vi "test-ElevatorSim-stability.vi"() -> (3 "Test Passed":bool)   [LabVIEW 2019]
uses:
  <vilib>/Rock Robotics/WPI/ThirdParty/JAS_Junk/TrajLib/TypeDef/DCMOTOR.CTL
  <vilib>/Rock Robotics/WPI/ThirdParty/JAS_Junk/TrajLib/TypeDef/ELEVATOR_SIM.ctl
  <vilib>/Rock Robotics/WPI/ThirdParty/JAS_Junk/TrajLib/TypeDef/LINEAR_SYSTEM_SIM.ctl
  <vilib>/Rock Robotics/WPI/ThirdParty/JAS_Junk/TrajLib/TypeDef/LINEAR_SYSTEM.ctl
  <vilib>/Analysis/Matrix/Datatypes/RealMatrix.ctl
  <vilib>/Rock Robotics/WPI/ThirdParty/JAS_Junk/TrajLib/MatBuilder_Create.vi
  <vilib>/Rock Robotics/WPI/ThirdParty/JAS_Junk/TrajLib/DCMotor_New.vi
  <vilib>/Rock Robotics/WPI/ThirdParty/JAS_Junk/TrajLib/VI/Units_RotationsPerMinuteToRadiansPerSecond.vi
  <vilib>/Rock Robotics/WPI/ThirdParty/JAS_Junk/TrajLib/Discretization_DiscretizeAB.vi
  <vilib>/Analysis/baseanly.llb/A x B.vi
  <vilib>/Analysis/baseanly.llb/Real A x B.vi
  <vilib>/Rock Robotics/WPI/ThirdParty/JAS_Junk/TrajLib/MatrixHelper_CoerceSize.vi
  <vilib>/Rock Robotics/WPI/ThirdParty/JAS_Junk/TrajLib/Matrix_Exp.vi
  <vilib>/Rock Robotics/WPI/ThirdParty/JAS_Junk/TrajLib/Matrix_AssignBlock.vi
  <vilib>/Rock Robotics/WPI/ThirdParty/JAS_Junk/TrajLib/Matrix_ExtractFrom.vi
  <vilib>/Analysis/7linalg.llb/Matrix Exp.vi
  <vilib>/Analysis/7linalg.llb/Real Matrix Exp.vi
  <vilib>/Analysis/Matrix/Numeric/Multiply/Multiply.vi
  <vilib>/Analysis/Matrix/Numeric/Multiply/Multiply - RM,R.vi
  <vilib>/Analysis/Matrix/Numeric/Add/Add.vi
  <vilib>/Analysis/Matrix/Numeric/Add/Add - RM,RM.vi
  <vilib>/Rock Robotics/WPI/ThirdParty/JAS_Junk/TrajLib/Trajectory_Library.lvlib
  <vilib>/Analysis/Matrix/NI_Matrix.lvlib
panel:
  in  "Tab Control":enum32{"Page 2", "Page 6", "Page 7"}(tab)
  out "Elevator Motor":T1 {"Jr_KgM2" format="%13.5p"; "L_H" format="%13.5p"; "Kt_NMPerAmp" format="%13.5p"; "KvINV_RadPerSecPerVolt" format="%13.5p"; "R_Ohms" format="%13.5p"; "FreeSpeed_RadPerSec" format="%13.5p"; "FreeCurrent_Amps" format="%13.5p"; "StallCurrent_Amps" format="%13.5p"; "StallTorque_NM" format="%13.5p"; "nominalVoltage_Volts" format="%13.5p"}
  out "Elevator Simulaation":T2={"LinearSystemSim"={"m_Plant"={"m_A"=[], "m_B"=[], "m_C"=[], "m_D"=[], "States"=0, "Inputs"=0, "Outputs"=0}, "m_X"=[], "m_Y"=[], "m_U"=[], "MeasureStdDev"=[]}, "GearBox"={"nominalVoltage_Volts"=0.0, "StallTorque_NM"=0.0, "StallCurrent_Amps"=0.0, "FreeCurrent_Amps"=0.0, "FreeSpeed_RadPerSec"=0.0, "R_Ohms"=0.0, "KvINV_RadPerSecPerVolt"=0.0, "Kt_NMPerAmp"=0.0, "L_H"=0.0, "Jr_KgM2"=0.0}, "Gearing"=0.0, "DrumRadius_M"=0.0, "MinHeight_M"=0.0, "MaxHeight_M"=0.0, "CarriageMass_Kg"=0.0, "SimulateGravity"=TRUE} {"GearBox"."Jr_KgM2" format="%13.5p"; "GearBox"."L_H" format="%13.5p"; "GearBox"."Kt_NMPerAmp" format="%13.5p"; "GearBox"."KvINV_RadPerSecPerVolt" format="%13.5p"; "GearBox"."R_Ohms" format="%13.5p"; "GearBox"."FreeSpeed_RadPerSec" format="%13.5p"; "GearBox"."FreeCurrent_Amps" format="%13.5p"; "GearBox"."StallCurrent_Amps" format="%13.5p"; "GearBox"."StallTorque_NM" format="%13.5p"; "GearBox"."nominalVoltage_Volts" format="%13.5p"}
  out "Velocity":cluster{"Voltage":dbl}(graph)
  out "PV Chart":cluster{dbl}(graph)
  out "At Top":bool
  out "At Bottom":bool
  out "Size Coerced":bool
  out "Alt Position Meters":dbl
  out "Position_Meters":dbl
  out "ApproxEquals":bool
  # "<States, 1>"
  # "<Outputs, 1>"
  # "<Inputs, 1>"
  # "<Outputs, 1>"
  # "<States,States>"
  # "<States,Inputs>"
  # "<Outputs,States>"
  # "<Outputs,Inputs>"
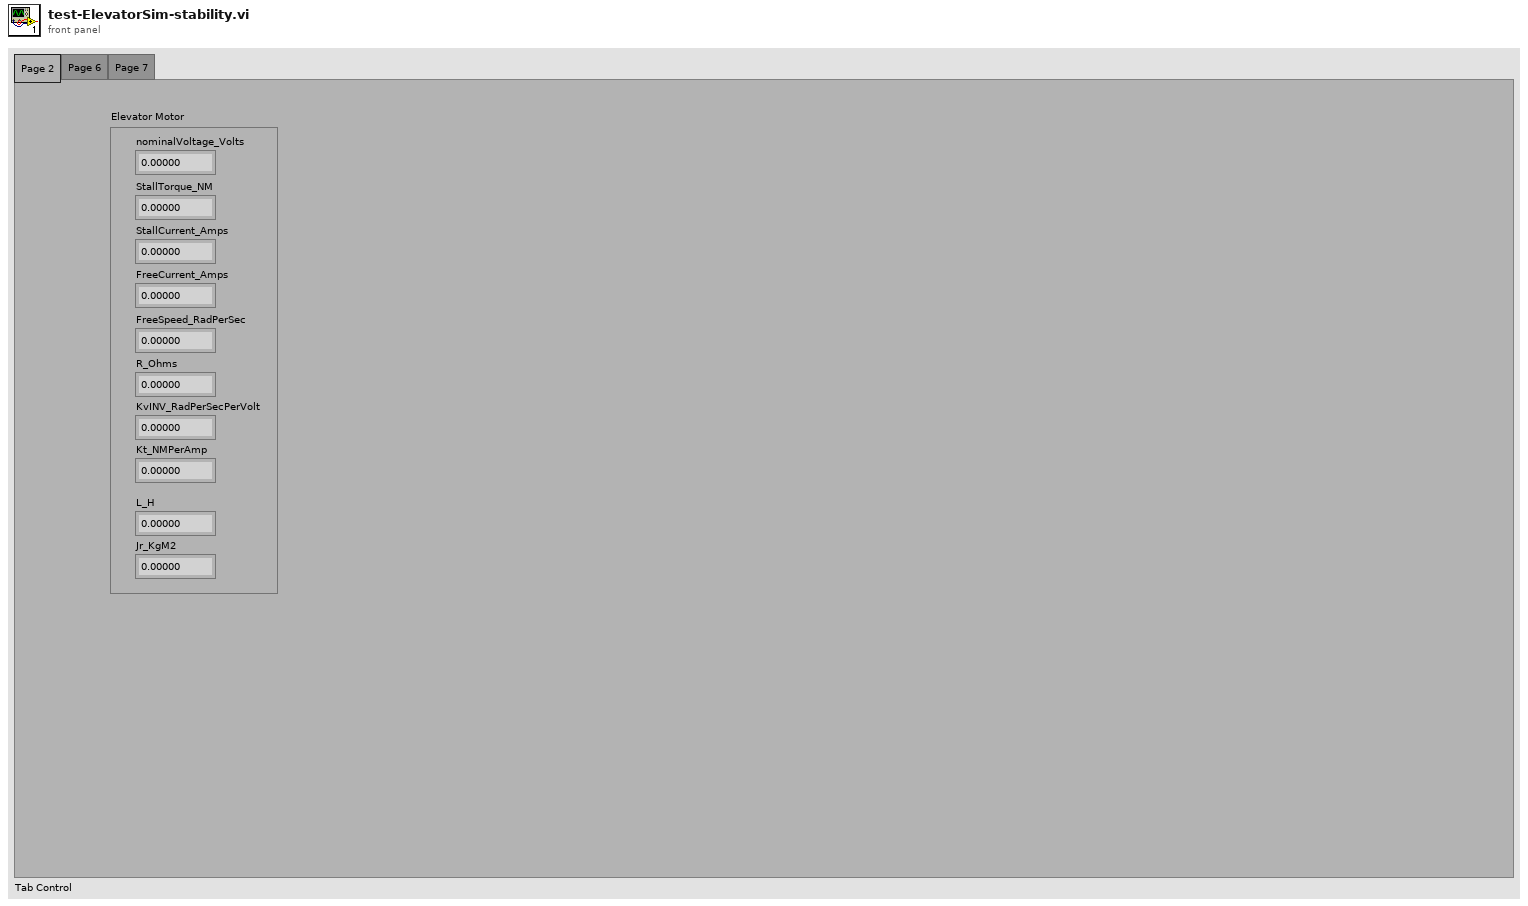
[diagram p1: front panel]
types:
  T1 = typedef "Trajectory_Library.lvlib/DCMOTOR.CTL" = cluster{"nominalVoltage_Volts":dbl, "StallTorque_NM":dbl, "StallCurrent_Amps":dbl, "FreeCurrent_Amps":dbl, "FreeSpeed_RadPerSec":dbl, "R_Ohms":dbl, "KvINV_RadPerSecPerVolt":dbl, "Kt_NMPerAmp":dbl, "L_H":dbl, "Jr_KgM2":dbl}
  T2 = typedef "Trajectory_Library.lvlib/ELEVATOR_SIM.ctl" = cluster{"LinearSystemSim":T3, "GearBox":T1, "Gearing":dbl, "DrumRadius_M":dbl, "MinHeight_M":dbl, "MaxHeight_M":dbl, "CarriageMass_Kg":dbl, "SimulateGravity":bool}
  T3 = typedef "Trajectory_Library.lvlib/LINEAR_SYSTEM_SIM.ctl" = cluster{"m_Plant":T4, "m_X":T5, "m_Y":T5, "m_U":T5, "MeasureStdDev":T5}
  T4 = typedef "Trajectory_Library.lvlib/LINEAR_SYSTEM.ctl" = cluster{"m_A":T5, "m_B":T5, "m_C":T5, "m_D":T5, "States":i32, "Inputs":i32, "Outputs":i32}
  T5 = typedef "NI_Matrix.lvlib/RealMatrix.ctl" = dbl[][]
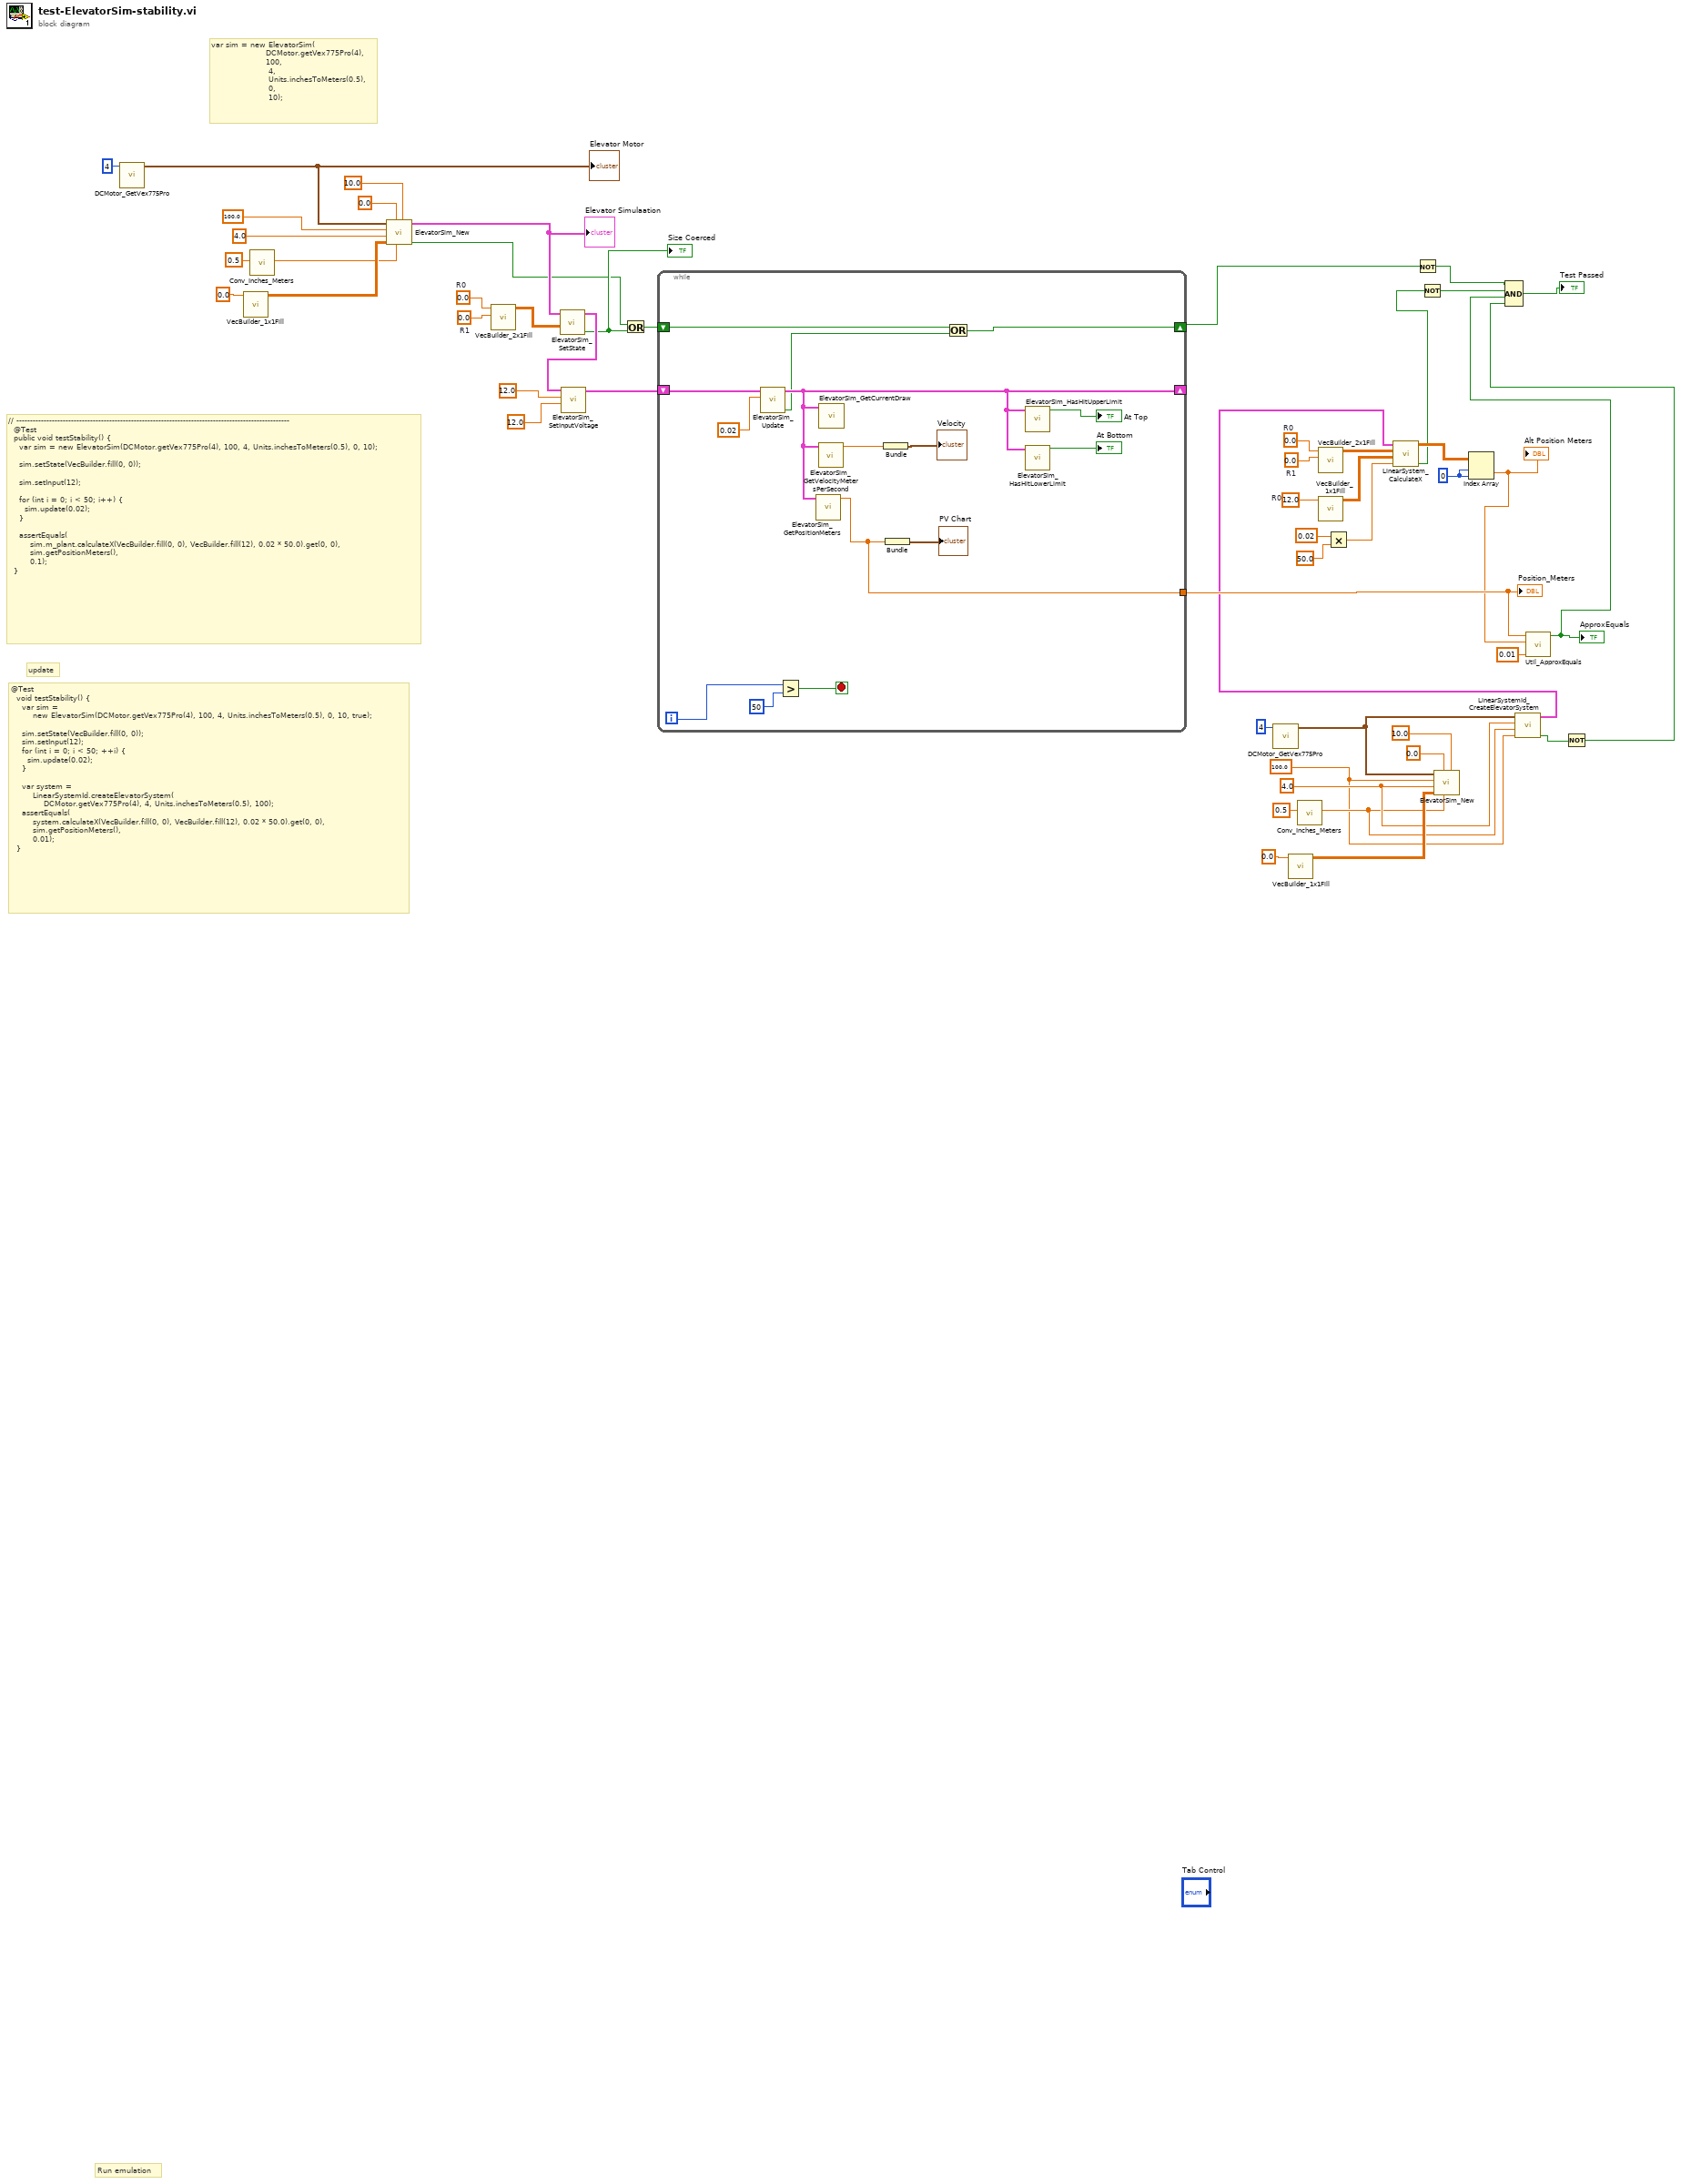
[diagram p0: block diagram]
diagram:
  w4 = 100.0 ("G")
  w6 = 4.0 ("massKg")
  w26 = 0 ("index (row)")
  w33 = 12.0  # R0
  w35 = 0.0  # R1
  w34 = 0.0  # R0
  w38 = 0.0  # R1
  w37 = 0.0  # R0
  # "update"
  # "@Test\n  void testStability() {\n    var sim =\n        new ElevatorSim(DCMotor.getVex775Pro(4), 100, 4, Units.inchesToMeters(0.5), 0, 10, true);\n\n    sim.setState(VecBuilder.fill(0, 0));\n    sim.setInput(12);\n    for (int i = 0; i < 50; ++i) {\n      sim.update(0.02);\n    }\n\n    var system =\n        LinearSystemId.createElevatorSystem(\n            DCMotor.getVex775Pro(4), 4, Units.inchesToMeters(0.5), 100);\n    assertEquals(\n        system.calculateX(VecBuilder.fill(0, 0), VecBuilder.fill(12), 0.02 * 50.0).get(0, 0),\n        sim.getPositionMeters(),\n        0.01);\n  }"
  # "// ----------------------------------------------------------------------------------------------------\n  @Test\n  public void testStability() {\n    var sim = new ElevatorSim(DCMotor.getVex775Pro(4), 100, 4, Units.inchesToMeters(0.5), 0, 10);\n\n    sim.setState(VecBuilder.fill(0, 0));\n\n    sim.setInput(12);\n\n    for (int i = 0; i < 50; i++) {\n      sim.update(0.02);\n    }\n\n    assertEquals(\n        sim.m_plant.calculateX(VecBuilder.fill(0, 0), VecBuilder.fill(12), 0.02 * 50.0).get(0, 0),\n        sim.getPositionMeters(),\n        0.1);\n  }"
  # "var sim = new ElevatorSim(\n                    DCMotor.getVex775Pro(4), \n                    100, \n                     4, \n                     Units.inchesToMeters(0.5), \n                     0, \n                     10);"
  # "Run emulation"
  n1 = call <vilib>:"DCMotor_GetVex775Pro.vi"("Num Motors"=4) -> ("DCMOTOR"=w46:T1)  [unwired: 10 in]
  "Elevator Motor" <- w46
  n2 = call <vilib>:"VecBuilder_1x1Fill.vi"("R0_C0"=0.0) -> ("output matrix"=w50:T5)  [unwired: 10 in]
  n3 = call <vilib>:"Conv_Inches_Meters.vi"("INCH"=0.5) -> ("Meters"=w44:dbl)  [unwired: 10 in]
  n4 = call <vilib>:"ElevatorSim_New.vi"("MaxHeight_Meters"=10.0, "DrumRadius_Meters"=w44, "MinHeight_Meters"=0.0, "MeasurementStdDev"=w50, "CarriageMass_Kg"=4.0 ("massKg"), "Gearing"=100.0 ("G"), "GearBox"=w46) -> ("Error"=w16:bool, "ElevatorSim"=w40:T2)  [unwired: 3 in]
  "Elevator Simulaation" <- w40
  n5 = call <vilib>:"VecBuilder_2x1Fill.vi"("R1"=w38, "R0"=w37) -> ("output matrix"=w36:T5)  [unwired: 9 in]
  n6 = call <vilib>:"ElevatorSim_SetState.vi"("System State"=w36, "in ElevatorSim"=w40) -> ("Size Coerced"=w17:bool, "out ElevatorSim"=w39:T2)  [unwired: 8 in]
  "Size Coerced" <- w17
  n7 = call <vilib>:"ElevatorSim_SetInputVoltage.vi"("Battery_Volts"=12.0, "Input_Voltage"=12.0, "in ElevatorSim"=w39) -> ("out ElevatorSim"=w41:T2)  [unwired: 8 in]
  n8 = Or(x=w16, y=w17) -> (x .or. y?=w18:bool)
  n9 = while {
    shift-right: [w62] -> _
    shift-left: w41 -> [w64]
    tunnel: [w57] -> w25
    shift-right: [w54] -> w15
    shift-left: w18 -> [w55]
    i -> [w60]
    stop <- w58 stop-if-true
    n10 = call <vilib>:"ElevatorSim_Update.vi"("dT_Seconds"=0.02, "in ElevatorSim"=w64) -> ("Error"=w56:bool, "out ElevatorSim"=w62:T2)  [unwired: 8 in]
    n11 = Greater?(x=w60, y=50) -> (0:w58:bool)
    n12 = call <vilib>:"ElevatorSim_GetPositionMeters.vi"("ElevatorSim"=w62) -> ("Position_Meters"=w57:dbl)  [unwired: 10 in]
    n13 = call <vilib>:"ElevatorSim_GetVelocityMetersPerSecond.vi"("ElevatorSim"=w62) -> ("Velocity_MetersPerSec"=w61:dbl)  [unwired: 10 in]
    n14 = call <vilib>:"ElevatorSim_GetCurrentDraw.vi"("ElevatorSim"=w62) -> ()  [unwired: 10 in, 1 out]
    n15 = Bundle("Velocity_MetersPerSec"=w61) -> (→"Velocity":cluster{"Velocity_MetersPerSec":dbl})  [unwired: 1 in]
    n16 = Bundle("Position_Meters"=w57) -> (→"PV Chart":cluster{"Position_Meters":dbl})  [unwired: 1 in]
    n17 = Or(x=w55, y=w56) -> (x .or. y?=w54:bool)
    n18 = call <vilib>:"ElevatorSim_HasHitUpperLimit.vi"("ElevatorSim"=w62) -> ("At HIgh LImit"=→"At Top":bool)  [unwired: 10 in]
    n19 = call <vilib>:"ElevatorSim_HasHitLowerLimit.vi"("ElevatorSim"=w62) -> ("AtLowLimit"=→"At Bottom":bool)  [unwired: 10 in]
  }
  "Position_Meters" <- w25
  n20 = call <vilib>:"DCMotor_GetVex775Pro.vi"("Num Motors"=4) -> ("DCMOTOR"=w7:T1)  [unwired: 10 in]
  n21 = call <vilib>:"VecBuilder_1x1Fill.vi"("R0_C0"=0.0) -> ("output matrix"=w10:T5)  [unwired: 10 in]
  n22 = call <vilib>:"Conv_Inches_Meters.vi"("INCH"=0.5) -> ("Meters"=w5:dbl)  [unwired: 10 in]
  n23 = call <vilib>:"VecBuilder_2x1Fill.vi"("R1"=w35, "R0"=w34) -> ("output matrix"=w32:T5)  [unwired: 9 in]
  n24 = call <vilib>:"VecBuilder_1x1Fill.vi"("R0_C0"=w33) -> ("output matrix"=w31:T5)  [unwired: 10 in]
  n25 = Multiply(x=0.02, y=50.0) -> (x*y=w28:dbl)
  n26 = Not(x=w15) -> (.not. x?=w14:bool)
  n27 = call <vilib>:"ElevatorSim_New.vi"("MaxHeight_Meters"=10.0, "DrumRadius_Meters"=w5, "MinHeight_Meters"=0.0, "MeasurementStdDev"=w10, "CarriageMass_Kg"=w6, "Gearing"=w4, "GearBox"=w7) -> ()  [unwired: 3 in, 2 out]
  n28 = call <vilib>:"LinearSystemId_CreateElevatorSystem.vi"("G"=w4, "radiusMeters"=w5, "massKg"=w6, "DCMOTOR"=w7) -> ("Size Coerced"=w2:bool, "Linearsystem"=w3:T4)  [unwired: 6 in]
  n29 = call <vilib>:"LinearSystem_CalculateX.vi"("dT_Seconds"=w28, "ClampedU"=w31, "X"=w32, "Linearsystem"=w3) -> ("Error"=w20:bool, "outX"=w27:T5)  [unwired: 6 in]
  n30 = Not(x=w20) -> (.not. x?=w19:bool)
  n31 = Index Array(array=w27, index (row)=w26, index (col)=w26) -> (element=w24:dbl)
  "Alt Position Meters" <- w24
  n32 = call <vilib>:"Util_ApproxEquals.vi"("Tolerance"=0.01, "Value 2"=w24, "Value 1"=w25) -> ("ApproxEquals"=w21:bool)  [unwired: 8 in]
  "ApproxEquals" <- w21
  n33 = Not(x=w2) -> (.not. x?=w1:bool)
  n34 = Compound Arithmetic op=AND(w14, w19, w21, w1) -> (→"Test Passed":bool)
